vi "Test002-pass.vi"() -> ()   [LabVIEW 2018]
uses:
  <vilib>/vision/NI_Vision_Development_Module.lvlib
panel:
  out "G 2":T1(plugin-control)
  in  "File Path 2":path=path "D:/Life/20191001_Accordance/Project/EPISIL/20200806-Camera/20200716/getimg_003.bmp"
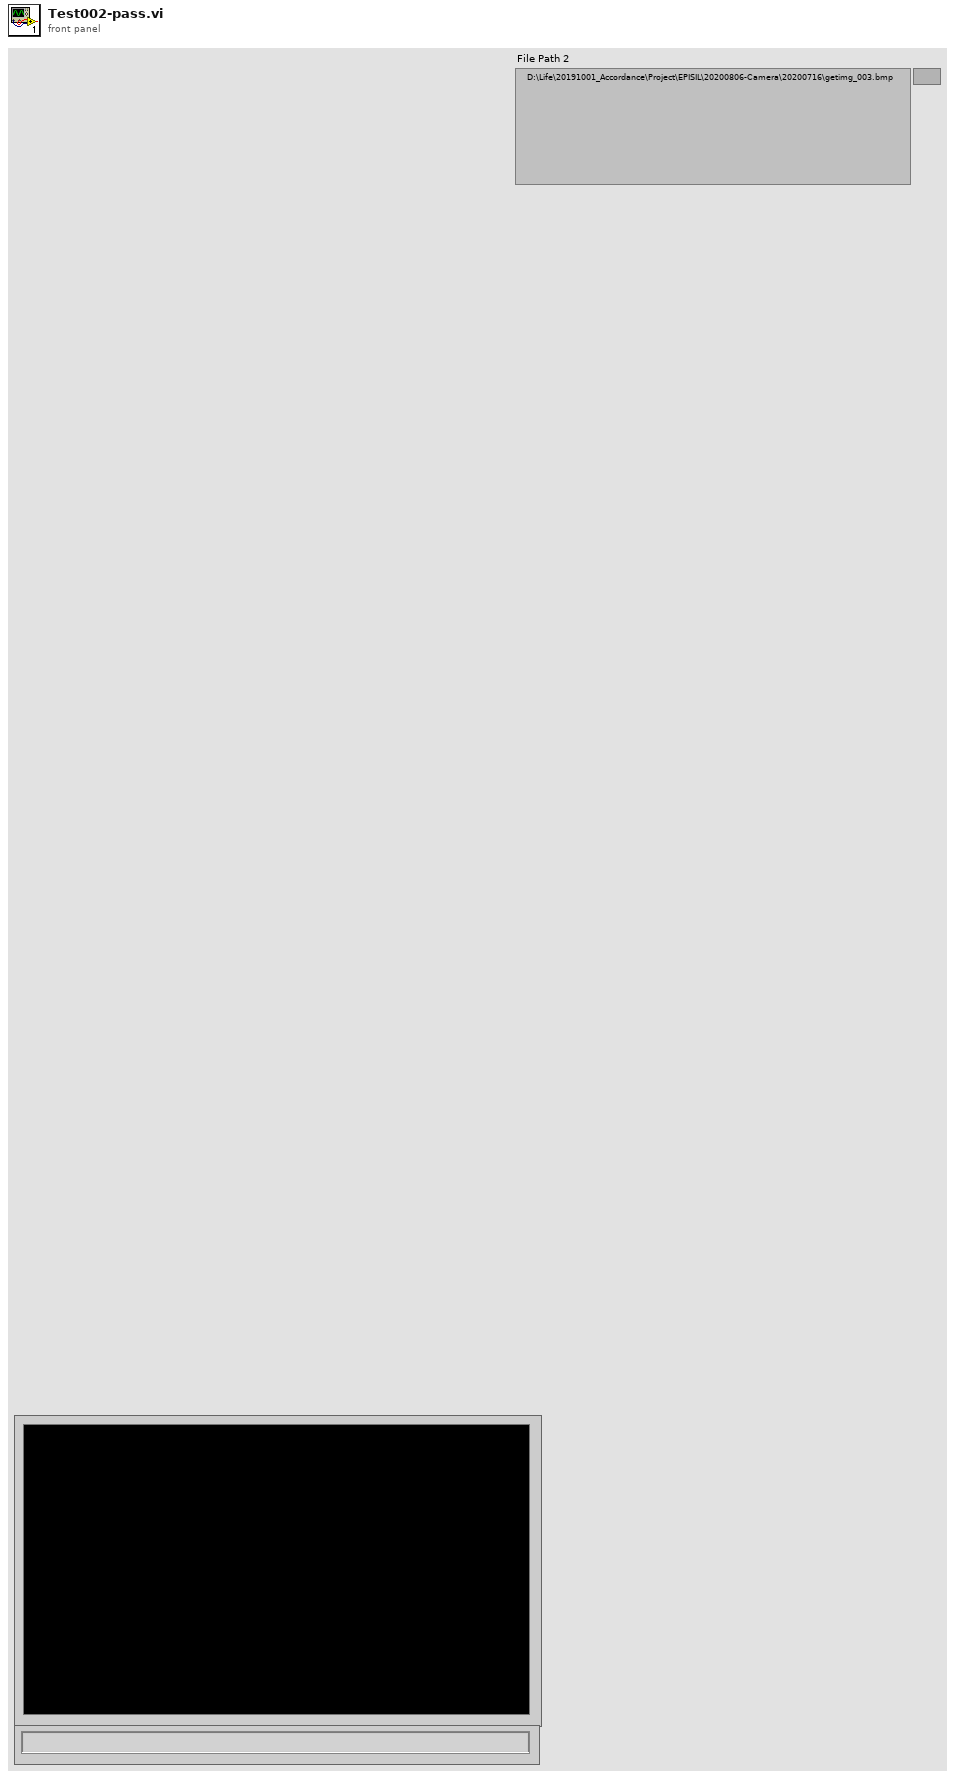
[diagram p1: front panel]
types:
  T1 = typedef "IMAQ Image.ctl" = refnum<image>
  T2 = typedef "Image Type" = u32
  T3 = typedef "IMAQ Rectangle" = cluster{"Left":i32, "Top":i32, "Right":i32, "Bottom":i32, "Rotation":dbl}
  T4 = cluster{"Left":i32, "Top":i32, "Right":i32, "Bottom":i32}
  T5 = typedef "ROI Descriptor" = cluster{"Global Rectangle":i32[], "Contours":cluster{"ID":enum32{"External", "Internal"}, "Type":u32, "Coordinates":i32[]}[]}
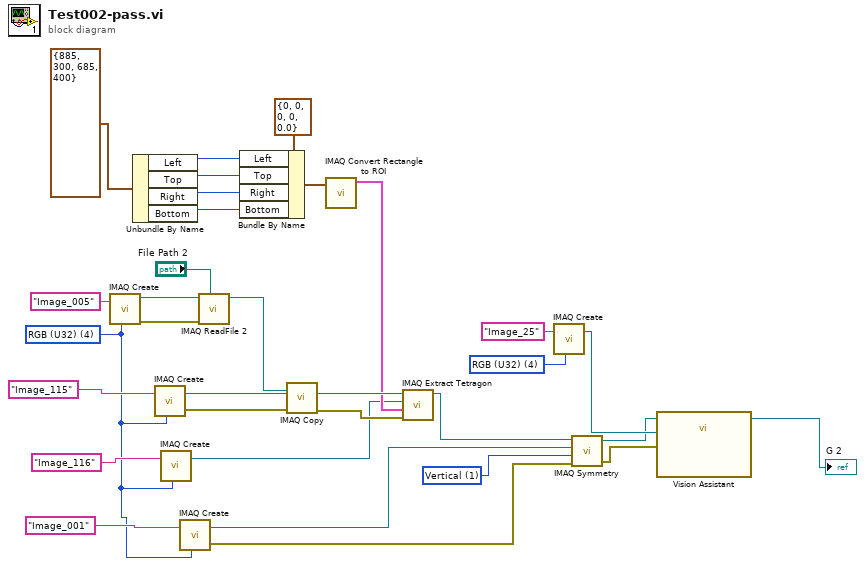
[diagram p0: block diagram]
diagram:
  w6 = T2 4 items=["Grayscale (U8)", "Grayscale (I16)", "Grayscale (SGL)", "Complex (CSG)", "RGB (U32)", "HSL (U32)", "RGB (U64)", "Grayscale (U16)"] ("Image Type")
  w8 = u32 1 items=["Horizontal", "Vertical", "Central", "1st Diagonal", "2nd Diagonal"] ("Type of Symmetry")
  w7 = T2 4 items=["Grayscale (U8)", "Grayscale (I16)", "Grayscale (SGL)", "Complex (CSG)", "RGB (U32)", "HSL (U32)", "RGB (U64)", "Grayscale (U16)"] ("Image Type")
  n1 = call "IMAQ Create"("Image Name"="Image_005", "Image Type"=w7) -> ("New Image"=w30:T1, "error out"=w31:errorcluster)  [unwired: 3 in]
  n2 = Unbundle By Name(T4 {"Left"=885, "Top"=300, "Right"=685, "Bottom"=400} ("Rectangle")) -> ("Left"=w14:i32, "Top"=w15:i32, "Right"=w16:i32, "Bottom"=w17:i32)
  n3 = call "IMAQ Create"("Image Name"="Image_115", "Image Type"=w7) -> ("New Image"=w21:T1, "error out"=w22:errorcluster)  [unwired: 3 in]
  n4 = call "IMAQ Create"("Image Name"="Image_116", "Image Type"=w7) -> ("New Image"=w9:T1)  [unwired: 3 in, 1 out]
  n5 = call "IMAQ Create"("Image Name"="Image_001", "Image Type"=w7) -> ("New Image"=w24:T1, "error out"=w23:errorcluster)  [unwired: 3 in]
  n6 = call "IMAQ ReadFile 2"("File Path"="File Path 2", "error in (no error)"=w31, "Image"=w30) -> ("Image Out"=w19:T1)  [unwired: 4 in, 4 out]
  n7 = Bundle By Name(cluster=T3 {"Left"=0, "Top"=0, "Right"=0, "Bottom"=0, "Rotation"=0.0} ("Rectangle"), "Left"=w14, "Top"=w15, "Right"=w16, "Bottom"=w17) -> (w18:T3)
  n8 = call "IMAQ Copy"("error in (no error)"=w22, "Image Dst"=w21, "Image Src"=w19) -> ("error out"=w28:errorcluster, "Image Dst Out"=w26:T1)  [unwired: 3 in]
  n9 = call "IMAQ Convert Rectangle to ROI"("Rectangle"=w18) -> ("ROI Descriptor"=w11:T5)  [unwired: 8 in, 1 out]
  n10 = call-poly "IMAQ Extract Tetragon"("error in (no error)"=w28, "ROI Descriptor"=w11, "Image Dst"=w9, "Image Src"=w26) -> ("Image Dst Out"=w27:T1)  [unwired: 6 in, 1 out]
  n11 = call "IMAQ Create"("Image Name"="Image_25", "Image Type"=w6) -> ("New Image"=w4:T1)  [unwired: 3 in, 1 out]
  n12 = call "IMAQ Symmetry"("error in (no error)"=w23, "Type of Symmetry"=w8, "Image Dst"=w24, "Image Src"=w27) -> ("error out"=w2:errorcluster, "Image Dst Out"=w3:T1)  [unwired: 1 in]
  n13 = call "Vision Assistant"("Image In"=w3, "Image Dst"=w4, "error in"=w2) -> ("Image Out"=→"G 2":T1)  [unwired: 23 in, 1 out]
